vi "dataset.set.vi"(8 "error in (no error)":errorcluster, 10 "datasources.lvlib:dataset.lvclass":refnum<class "dataset.lvclass">, 11 "target in":refnum<class "target.lvclass">) -> (0 "error out":errorcluster, 3 "target out":refnum<class "target.lvclass">)   [LabVIEW 2020, in "datasources.lvlib" / "target.lvclass"]
uses:
  target.lvclass
  dataset/dataset.lvclass
  target.lvclass/target.ctl
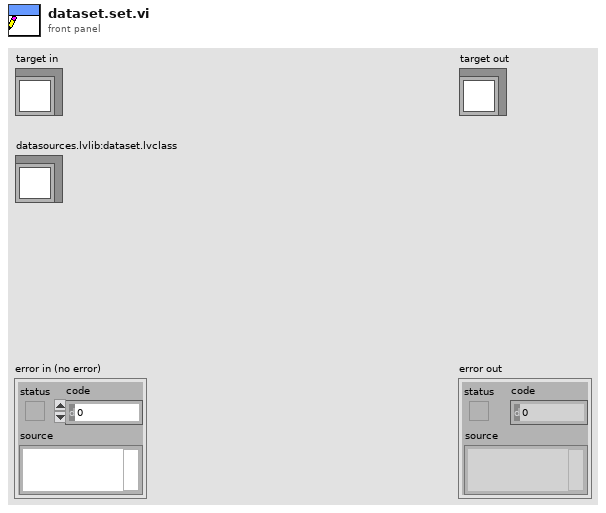
[diagram p1: front panel]
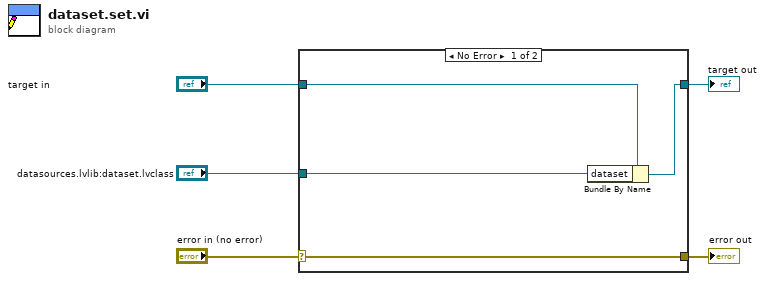
[diagram p0: block diagram]
diagram:
  n1 = case shown="No Error" "error in (no error)" {
    selector: "error in (no error)" -> [w9 w10]
    tunnel: [w9 w10] -> w4
    tunnel: [w7 w11] -> w2
    tunnel: "target in" -> [w8 w11]
    tunnel: "datasources.lvlib:dataset.lvclass" -> [w6 _]
    frame No Error {
      n2 = Bundle By Name(cluster=w8, "dataset"=w6) -> (w7:refnum<class "target.lvclass">)
    }
    frame Error {
    }
  }
  "error out" <- w4
  "target out" <- w2
